vi "Startup Lockin.vi"(11 "Hardware Parameters In":T2={"Scan Calibration [G/V]"=0.0, "Modulation Calibration [G/V]"=0.0, "Modulation Phase [deg]"=0.0, "Modulation Frequency [Hz]"=0.0, "Attenuation [dB]"=0, "Input Channel Count"=0, "Time constant"=7, "Sensitivity"=17, "Frequency Output Voltage [V]"=0.0, "Phase Output Voltage [V]"=0.0, "Lock-in Offset Compensation"=FALSE, "RF [GHz]"=0.0, "Q Start"=0.0, "Q End"=0.0, "Balance"=0.0, "Phase Error"=0.0, "AFC Error"=0.0, "AFC"=FALSE, "Magnet Rotation"=FALSE, "Balance Scaling Factor"=1.0, "Phase Error Scaling Factor"=1.0, "AFC Error Scaling Factor"=1.0, "Frequency Counter ID"="", "Sweep Waveform"=enum."Sawtooth", "Q-Factor Scale"=0.0, " Q-Data Scale"=0.0, " Q-Data Offset"=0.0, "Magnet Rotation Slope"=0.0, "Magnet Rotation Offset"=0.0, "Phase Sweep Resolution"=0.0, "Hardware Version Number"="", "Spectrometer ID Number"=0, "Spectrometer Name"="", "Lock in Saturation"=0.0, "Balance Threshold"=0.0, "Phase Error Threshold"=0.0, "AFC Error Threshold"=0.0, "Linear Actuator Length"=0.0, "Lock-in OK?"=FALSE, "Ignore Lock-in Comm. Failure"=FALSE, "Gradient Addresses"=[], "Gradient Calibrations [G/A*mm]"=[], "Gradient Power Supplies"=[], "Lock-in Address"="", "Magnet Type"=enum."RRI", "Camera Names"=[], "Sweep Limit [Gauss]"=0.0, "Modulation Limit [Gauss]"=0.0, "Balance Threshold Exceeded?"=FALSE, "Phase Threshold Exceeded?"=FALSE, "AFC Threshold Exceeded?"=FALSE, "Consecutive Re-tune attempts"=0, "Reverse Sweep Slope [sec]"=0.0, "Reverse Sweep Offset [G]"=0.0, "AFC Field Correction [V/MHz]"=0.0, "Active Gradients (X Y Z)"=[], "SpO2 Calibration [SpO2/V]"=1.0, "Heart Rate Calibration [BPM/V]"=1.0, "Thermocouple Channel"=""} {"Sensitivity" items=["", "2 nV", "5 nV", "10 nV", "20 nV", "50 nV", "100 nV", "200 nV", "500 nV", "1 uV", "2 uV", "5 uV", "10 uV", "20 uV", "50 uV", "100 uV", "200 uV", "500 uV", "1 mV", "2 mV", "5 mV", "10 mV", "20 mV", "50 mV", "100 mV", "200 mV", "500 mV", "1 V"]; "Time constant" items=["10 us", "20 us", "40 us", "80 us", "160 us", "320 us", "640 us", "5 ms", "10 ms", "20 ms", "50 ms", "100 ms", "200 ms", "500 ms", "1 s", "2 s", "5 s", "10 s", "20 s", "50 s", "100 s", "200 s", "500 s", "1 ks", "2 ks", "5 ks", "10 ks", "20 ks", "50 ks", "100 ks"]}) -> (0 "error out":errorcluster, 1 "QSM Response":cluster{"Enum":T1, "Data":variant}[](array[cluster]), 2 "Lockin OK?":bool, 3 "Hardware Parameters Out":T2={"Scan Calibration [G/V]"=0.0, "Modulation Calibration [G/V]"=0.0, "Modulation Phase [deg]"=0.0, "Modulation Frequency [Hz]"=0.0, "Attenuation [dB]"=0, "Input Channel Count"=0, "Time constant"=7, "Sensitivity"=17, "Frequency Output Voltage [V]"=0.0, "Phase Output Voltage [V]"=0.0, "Lock-in Offset Compensation"=FALSE, "RF [GHz]"=0.0, "Q Start"=0.0, "Q End"=0.0, "Balance"=0.0, "Phase Error"=0.0, "AFC Error"=0.0, "AFC"=FALSE, "Magnet Rotation"=FALSE, "Balance Scaling Factor"=1.0, "Phase Error Scaling Factor"=1.0, "AFC Error Scaling Factor"=1.0, "Frequency Counter ID"="", "Sweep Waveform"=enum."Sawtooth", "Q-Factor Scale"=0.0, " Q-Data Scale"=0.0, " Q-Data Offset"=0.0, "Magnet Rotation Slope"=0.0, "Magnet Rotation Offset"=0.0, "Phase Sweep Resolution"=0.0, "Hardware Version Number"="", "Spectrometer ID Number"=0, "Spectrometer Name"="", "Lock in Saturation"=0.0, "Balance Threshold"=0.0, "Phase Error Threshold"=0.0, "AFC Error Threshold"=0.0, "Linear Actuator Length"=0.0, "Lock-in OK?"=FALSE, "Ignore Lock-in Comm. Failure"=FALSE, "Gradient Addresses"=[], "Gradient Calibrations [G/A*mm]"=[], "Gradient Power Supplies"=[], "Lock-in Address"="", "Magnet Type"=enum."RRI", "Camera Names"=[], "Sweep Limit [Gauss]"=0.0, "Modulation Limit [Gauss]"=0.0, "Balance Threshold Exceeded?"=FALSE, "Phase Threshold Exceeded?"=FALSE, "AFC Threshold Exceeded?"=FALSE, "Consecutive Re-tune attempts"=0, "Reverse Sweep Slope [sec]"=0.0, "Reverse Sweep Offset [G]"=0.0, "AFC Field Correction [V/MHz]"=0.0, "Active Gradients (X Y Z)"=[], "SpO2 Calibration [SpO2/V]"=1.0, "Heart Rate Calibration [BPM/V]"=1.0, "Thermocouple Channel"=""} {"Sensitivity" items=["", "2 nV", "5 nV", "10 nV", "20 nV", "50 nV", "100 nV", "200 nV", "500 nV", "1 uV", "2 uV", "5 uV", "10 uV", "20 uV", "50 uV", "100 uV", "200 uV", "500 uV", "1 mV", "2 mV", "5 mV", "10 mV", "20 mV", "50 mV", "100 mV", "200 mV", "500 mV", "1 V"]; "Time constant" items=["10 us", "20 us", "40 us", "80 us", "160 us", "320 us", "640 us", "5 ms", "10 ms", "20 ms", "50 ms", "100 ms", "200 ms", "500 ms", "1 s", "2 s", "5 s", "10 s", "20 s", "50 s", "100 s", "200 s", "500 s", "1 ks", "2 ks", "5 ks", "10 ks", "20 ks", "50 ks", "100 ks"]})   [LabVIEW 2016]
uses:
  Types/Hardware Parameters.ctl
  Types/State Control.ctl
panel:
  # "Bridge I/O"
  # "Magnet Rotation"
  # "Field Calibration"
  # "Lock In Amplifier"
  # "Spectrometer Information"
  # "DAQ Settings"
  # "Gradient Coils and Field"
  # "X"
  # "Y"
  # "Z"
  # "Q-Measurements"
  # "Bridge I/O"
  # "Magnet Rotation"
  # "Field Calibration"
  # "Lock In Amplifier"
  # "Spectrometer Information"
  # "DAQ Settings"
  # "Gradient Coils and Field"
  # "X"
  # "Y"
  # "Z"
  # "Q-Measurements"
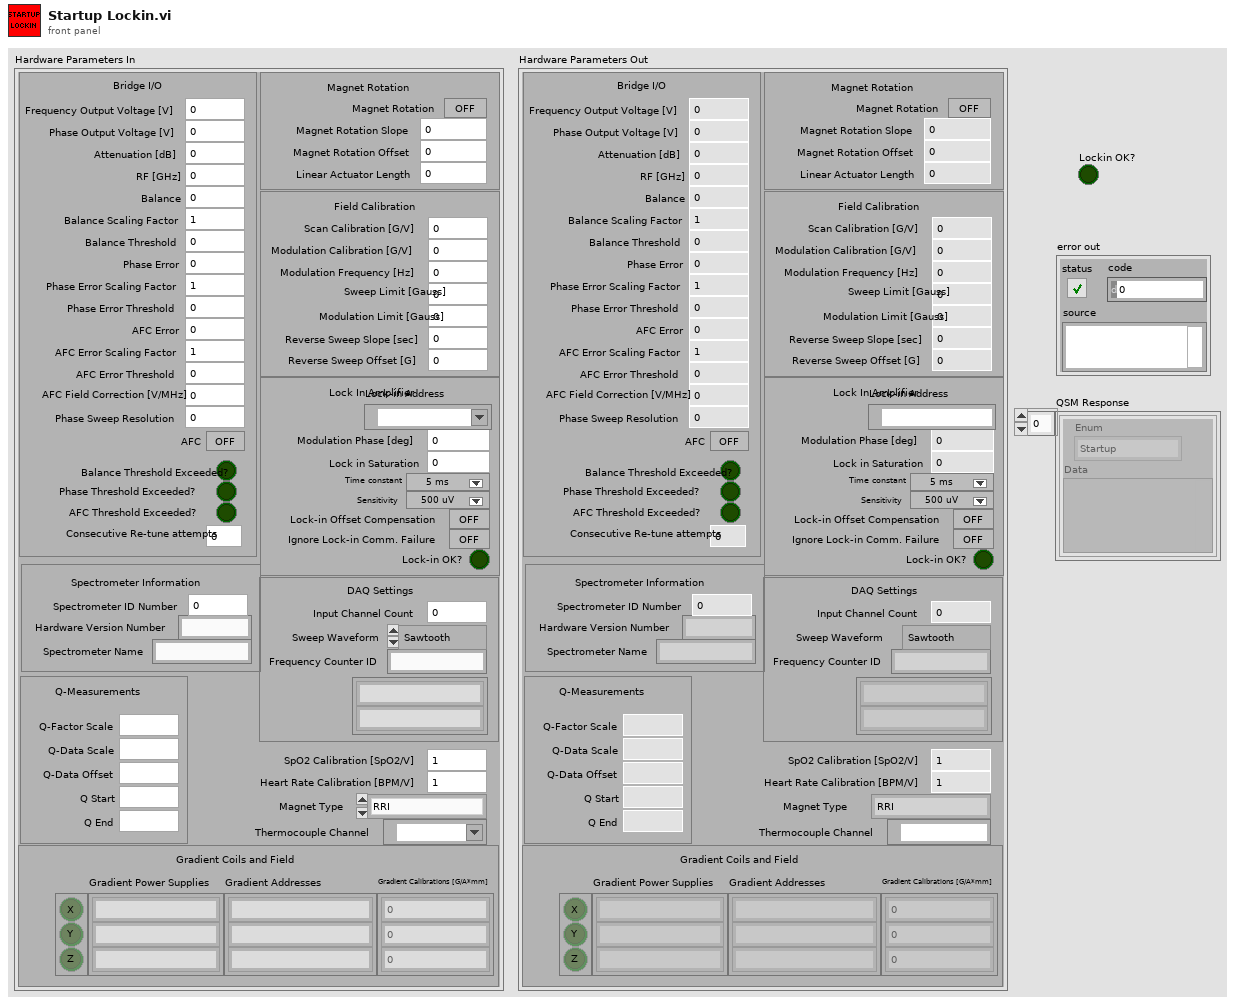
[diagram p1: front panel]
types:
  T1 = typedef "State Control.ctl" = enum16{"Startup", "Read Config File", "Initilize Optional Hardware", "Idle", "New Session", "Read GUI Pars", "Configure Hardware", "Initialize Set", "Pre-Scan", "Scan", "Post-Scan", "Exit Set", "Automated Tuning", "Manual Tuning", "Check Calibration", "Optimize RF Power", "Test Scan", "Set Oxy QA-Scan Pars", "Find Peaks", "Update from Cursors", "Flag Bad Set", "Mark transition time", "Measure Q", "Measure Noise", "Rotate Magnet", "Lock Field", "Engineering Tuning", "Zero Voltages", "Update Center Field", "Refit Data", "Open Session Data Folder", "AfterSave", "Undo Auto Update Pars", "Read from Script", "End Session", "Quit Software", "Error"}
  T2 = typedef "Hardware Parameters.ctl" = cluster{"Scan Calibration [G/V]":dbl, "Modulation Calibration [G/V]":dbl, "Modulation Phase [deg]":dbl, "Modulation Frequency [Hz]":dbl, "Attenuation [dB]":u16, "Input Channel Count":i32, "Time constant":u16, "Sensitivity":u16, "Frequency Output Voltage [V]":dbl, "Phase Output Voltage [V]":dbl, "Lock-in Offset Compensation":bool, "RF [GHz]":dbl, "Q Start":dbl, "Q End":dbl, "Balance":dbl, "Phase Error":dbl, "AFC Error":dbl, "AFC":bool, "Magnet Rotation":bool, "Balance Scaling Factor":dbl, "Phase Error Scaling Factor":dbl, "AFC Error Scaling Factor":dbl, "Frequency Counter ID":string, "Sweep Waveform":enum16{"Sine Wave", "Square Wave", "Sawtooth", "Triangle Wave"}, "Q-Factor Scale":dbl, " Q-Data Scale":dbl, " Q-Data Offset":dbl, "Magnet Rotation Slope":dbl, "Magnet Rotation Offset":dbl, "Phase Sweep Resolution":dbl, "Hardware Version Number":string, "Spectrometer ID Number":i32, "Spectrometer Name":string, "Lock in Saturation":dbl, "Balance Threshold":dbl, "Phase Error Threshold":dbl, "AFC Error Threshold":dbl, "Linear Actuator Length":dbl, "Lock-in OK?":bool, "Ignore Lock-in Comm. Failure":bool, "Gradient Addresses":string[], "Gradient Calibrations [G/A*mm]":dbl[], "Gradient Power Supplies":string[], "Lock-in Address":refnum<visa-resource-name>, "Magnet Type":enum16{"RRI", "BARDA", "Whole Body Permanent", "RRI Electromagnet"}, "Camera Names":string[], "Sweep Limit [Gauss]":dbl, "Modulation Limit [Gauss]":dbl, "Balance Threshold Exceeded?":bool, "Phase Threshold Exceeded?":bool, "AFC Threshold Exceeded?":bool, "Consecutive Re-tune attempts":i32, "Reverse Sweep Slope [sec]":dbl, "Reverse Sweep Offset [G]":dbl, "AFC Field Correction [V/MHz]":dbl, "Active Gradients (X Y Z)":bool[], "SpO2 Calibration [SpO2/V]":dbl, "Heart Rate Calibration [BPM/V]":dbl, "Thermocouple Channel":tag}
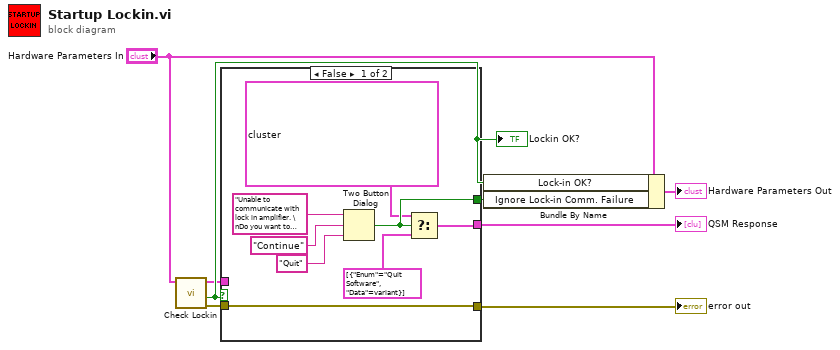
[diagram p0: block diagram]
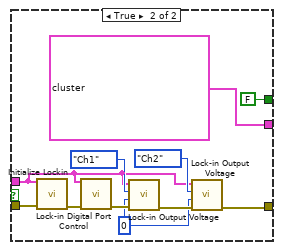
[diagram p2: hidden frame]
diagram:
  n1 = call "Check Lockin.vi"("Hardware Parameters"="Hardware Parameters In") -> ("error out"=w3:errorcluster, "Lockin OK?"=w8:bool, "Hardware Parameters Out"=w7:T2)  [unwired: 8 in]
  "Lockin OK?" <- w8
  n2 = case shown="False" w8 {
    tunnel: w3 -> [w11 w27]
    tunnel: [w11 w20] -> w6
    tunnel: [w12 cluster{"Enum":T1, "Data":variant}[] [{"Enum"=enum."Read Config File", "Data"=variant}, {"Enum"=enum."Configure Hardware", "Data"=variant}, {"Enum"=enum."Initilize Optional Hardware", "Data"=variant}, {"Enum"=enum."Idle", "Data"=variant}]] -> w5
    tunnel: [w10 FALSE ("T button?")] -> w4
    tunnel: w7 -> [_ w17]
    frame False {
      n3 = Two Button Dialog(message="Unable to communicate with lock in amplifier. \nDo you want to continue, or quit the software?", 1:"Quit" ("F button name (\"Cancel\")"), 2:"Continue" ("T button name (\"OK\")")) -> (T button?=w10:bool)
      n4 = Select(t=cluster{"Enum":T1, "Data":variant}[] [{"Enum"=enum."Read Config File", "Data"=variant}, {"Enum"=enum."Configure Hardware", "Data"=variant}, {"Enum"=enum."Initilize Optional Hardware", "Data"=variant}, {"Enum"=enum."Idle", "Data"=variant}], s=w10, f=cluster{"Enum":T1, "Data":variant}[] [{"Enum"=enum."Quit Software", "Data"=variant}]) -> (s? t:f=w12:cluster{"Enum":T1, "Data":variant}[])
    }
    frame True {
      w18 = 0 ("Output Voltage [V]")
      n5 = call "Initialize Lockin.vi"("error in (no error)"=w27, "Hardware Parameters"=w17) -> ("error out"=w24:errorcluster)  [unwired: 9 in]
      n6 = call "Lock-in Digital Port Control.vi"("error in (no error)"=w24, "Hardware Parameters"=w17) -> ("error out"=w23:errorcluster)  [unwired: 9 in]
      n7 = call "Lock-in Output Voltage.vi"("error in (no error)"=w23, "Output Voltage [V]"=w18, "Output Channel"=enum16{"Ch1", "Ch2"}."Ch1", "Hardware Parameters"=w17) -> ("error out"=w21:errorcluster)  [unwired: 7 in]
      n8 = call "Lock-in Output Voltage.vi"("error in (no error)"=w21, "Output Voltage [V]"=w18, "Output Channel"=enum16{"Ch1", "Ch2"}."Ch2", "Hardware Parameters"=w17) -> ("error out"=w20:errorcluster)  [unwired: 7 in]
    }
  }
  "QSM Response" <- w5
  "error out" <- w6
  n9 = Bundle By Name(cluster="Hardware Parameters In", "Lock-in OK?"=w8, "Ignore Lock-in Comm. Failure"=w4) -> (→"Hardware Parameters Out":T2)
